vi "UHR-Fleezers Control (host) - Lorentz v4.vi"() -> ()   [LabVIEW 2014] (continued)
                n3907 = Array Subset(array=w6030, index=w5984, length="N pts to average") -> (w6046:dbl[])
                n3908 = Array Subset(array=w6025, index=w5983, length="N pts to average") -> (w6028:dbl[])
                n3909 = Array Subset(array=w6025, index=w5984, length="N pts to average") -> (w6027:dbl[])
                n3910 = Array Subset(array=w5986, index=w5983, length="N pts to average") -> (w5995:dbl[])
                n3911 = Array Subset(array=w5986, index=w5984, length="N pts to average") -> (w5994:dbl[])
                n3912 = Index Array(array=w6008, index=0) -> (element=w6006:waveform(dbl))
                n3913 = call-poly <vilib>:"Mean.vi"("X"=w6047) -> ("mean"=w6045:dbl)  [unwired: 1 out]
                n3914 = call-poly <vilib>:"Mean.vi"("X"=w6028) -> ("mean"=w6024:dbl)  [unwired: 1 out]
                n3915 = call-poly <vilib>:"Mean.vi"("X"=w6046) -> ("mean"=w6044:dbl)  [unwired: 1 out]
                n3916 = call-poly <vilib>:"Mean.vi"("X"=w6027) -> ("mean"=w6023:dbl)  [unwired: 1 out]
                n3917 = call-poly <vilib>:"Mean.vi"("X"=w5995) -> ("mean"=w5993:dbl)  [unwired: 1 out]
                n3918 = call-poly <vilib>:"Mean.vi"("X"=w5994) -> ("mean"=w5992:dbl)  [unwired: 1 out]
                n3919 = Unbundle By Name(w6006) -> ("Y"=w6004:dbl[])
                n3920 = Subtract(x=w6024, y=w6023) -> (x-y=w6015:dbl)
                "Delta Fl. 2" <- w6015
                n3921 = Subtract(x=w5993, y=w5992) -> (x-y=w5987:dbl)
                "Delta Fl. 3" <- w5987
                n3922 = Subtract(x=w6045, y=w6044) -> (x-y=w6042:dbl)
                "Delta Fl. 1" <- w6042
                n3923 = feedback #34(w6004) -> (w6003:dbl[])
                n3924 = Build Array (concatenate)(w6003, w6004) -> (w6005:dbl[])
                n3925 = Initialize Array(w6042, 1 ("dimension size")) -> (w6039:dbl[])
                n3926 = Initialize Array(w6015, 1 ("dimension size")) -> (w6020:dbl[])
                n3927 = Initialize Array(w5987, 1 ("dimension size")) -> (w5989:dbl[])
                n3928 = Select(t=w6004, s=w5975, f=w6005) -> (s? t:f=w6002:dbl[])
                "Saved trap pos" <- w6002
                n3929 = feedback-in #34(w6002) -> ()
                n3930 = feedback #35(w6039) -> (w6040:dbl[])
                n3931 = Build Array (concatenate)(w6040, w6039) -> (w6038:dbl[])
                n3932 = feedback #36(w6020) -> (w6021:dbl[])
                n3933 = feedback #37(w5989) -> (w5990:dbl[])
                n3934 = Build Array (concatenate)(w6021, w6020) -> (w6019:dbl[])
                n3935 = Build Array (concatenate)(w5990, w5989) -> (w5988:dbl[])
                n3936 = Select(t=w6039, s=w5975, f=w6038) -> (s? t:f=w6018:dbl[])
                n3937 = feedback-in #35(w6018) -> ()
                n3938 = Select(t=w6020, s=w5975, f=w6019) -> (s? t:f=w6017:dbl[])
                n3939 = feedback-in #36(w6017) -> ()
                n3940 = Select(t=w5989, s=w5975, f=w5988) -> (s? t:f=w5982:dbl[])
                n3941 = feedback-in #37(w5982) -> ()
                n3942 = Build Array(w6018, w6017, w5982) -> (→"Save APD Deriv":dbl[][])
                n3943 = Index Array(array=w5974, index=15) -> (element=w5980:waveform(dbl))
                n3944 = Unbundle By Name(w5980) -> ("Y"=w5978:dbl[])
                n3945 = feedback #38(w5978) -> (w5977:dbl[])
                n3946 = Build Array (concatenate)(w5977, w5978) -> (w5979:dbl[])
                n3947 = Select(t=w5978, s=w5975, f=w5979) -> (s? t:f=w5976:dbl[])
                "Amp current" <- w5976
                n3948 = feedback-in #38(w5976) -> ()
              }
            }
            "Progress" <- w5951
            "Progress 2" <- w5951
          }
        }
      }
    }
    n3949 = local read "wait to reset values"() -> (w4817:bool)
    n3950 = Not(x=w4815) -> (.not. x?=w4818:bool)
    n3951 = And(x=w4818, y=w4817) -> (x .and. y?=w4819:bool)
    n3952 = case "Part of MCL raster scanning: returns to initial positions after scan done" shown="True" w4819 {
      tunnel: w4565 -> [w5414 w5421]
      tunnel: [w5414 w5420] -> w4821
      tunnel: w4666 -> [w5413 w5419]
      tunnel: [w5413 w5418] -> w4816
      frame False {
      }
      frame True {
        w5429 = 10.0 ("y")
        w5428 = 32767.0 ("y")
        # "to return scan values\nafter a synchronous \nAOM scan"
        n3953 = local read "AO2"() -> (w5422:dbl)
        n3954 = local read "AO1"() -> (w5423:dbl)
        n3955 = local write "wait to reset values"(FALSE ("wait to reset values")) -> ()
        n3956 = Multiply(x=w5423, y=w5428) -> (x*y=w5425:dbl)
        n3957 = Multiply(x=w5422, y=w5428) -> (x*y=w5427:dbl)
        n3958 = Divide(x=w5425, y=w5429) -> (x/y=w5424:dbl)
        n3959 = Divide(x=w5427, y=w5429) -> (x/y=w5426:dbl)
        n3960 = To Word Integer(number=w5424) -> (16bit integer=w5430:i16)
        n3961 = To Word Integer(number=w5426) -> (16bit integer=w5431:i16)
        n3962 = local read "Total Counts (ticks)"() -> (w5415:u16)
        n3963 = local read "Scan Range (V)\n(of steps)"() -> (w5416:dbl)
        n3964 = xnode "Read/Write Control"("FPGA VI Reference In"=w5421, "error in"=w5419, "AO1"=w5430, "AO2"=w5431, "MCL count"=w5415) -> ("FPGA VI Reference Out"=w5420:T50, "error out"=w5418:errorcluster)
        n3965 = property on="Scan Range (V)\n(of steps)" class="DigNum (strict)"("Val(Sgnl)"=w5416) -> ()  [unwired: 2 in, 2 out]
      }
    }
    n3966 = case shown="True" "Sound ON" {
      tunnel: [w4934 w4979] -> w4618
      tunnel: w4617 -> [w4934 w4978]
      tunnel: w4615 -> [_ _]
      tunnel: w4594 -> [_ w4937]
      tunnel: w4614 -> [_ _]
      tunnel: w4613 -> [_ w4948]
      tunnel: w4612 -> [_ w4958]
      frame False {
      }
      frame True {
        n3967 = Index Array(array=w4937, index="Data channel to sound") -> (element=w4936:waveform(dbl))
        "Waveform Graph 2" <- w4936
        n3968 = Unbundle By Name(w4936) -> ("dt"=w4962:dbl, "Y"=w4960:dbl[])
        n3969 = Array Size(array=w4960) -> (size(s)=w4961:i32)
        "N data samples" <- w4961
        n3970 = for "Data time base" {
          N: w4961 -> [_]
          tunnel: [w4983] -> w4963 mode=indexing
          i -> [w4983]
        }
        n3971 = Multiply(x=w4962, y=w4963) -> (x*y=w4959:dbl[])
        n3972 = Compound Arithmetic op=MULTIPLY(6.283185307179586, "Carrier Frequency (Hz)", w4958) -> (w4975:dbl[])
        n3973 = call <vilib>:"Interpolate 1D.vi"("X is monotonic"=TRUE, "xi"=w4958, "X"=w4959, "Y"=w4960) -> ("yi"=w4956:dbl[])  [unwired: 5 in, 2 out]
        n3974 = Sine(x=w4975) -> (sin(x)=w4964:dbl[])
        n3975 = Add(x=w4956, y="Offset") -> (x+y=w4954:dbl[])
        n3976 = Multiply(x=w4954, y="mult x") -> (x*y=w4952:dbl[])
        n3977 = Add(x="Offset 2", y=w4952) -> (x+y=w4947:dbl[])
        n3978 = Compound Arithmetic op=MULTIPLY(6.283185307179586, "Carrier Frequency (Hz)", w4948, w4947) -> (w4939:dbl[])
        n3979 = for "Cumulative sum" {
          tunnel: [w4982] -> w4945 mode=indexing
          shift-right: [w4982] -> w4942
          shift-left: 0.0 -> [w4981]
          tunnel: w4939 -> [w4980] mode=indexing
          n3980 = Add(x=w4980, y=w4981) -> (x+y=w4982:dbl)
        }
        n3981 = feedback #39(0.0) -> (w4941:dbl)
        n3982 = Add(x=w4945, y=w4941) -> (x+y=w4944:dbl[])
        n3983 = Add(x=w4942, y=w4941) -> (x+y=w4940:dbl)
        n3984 = feedback-in #39(w4940) -> ()
        n3985 = Sine(x=w4944) -> (sin(x)=w4938:dbl[])
        n3986 = Select(t=w4964, s="tone or data", f=w4938) -> (s? t:f=w4970:dbl[])
        n3987 = Multiply(x=w4970, y="Volume") -> (x*y=w4968:dbl[])
        n3988 = Initialize Array(0.0 ("element"), "N initial buffer elements") -> (w4971:dbl[])
        n3989 = Multiply(x="N initial buffer elements", y=w4948) -> (x*y=→"Initial buffer time (s)":dbl)
        n3990 = Build Array (concatenate)(w4971, w4968) -> (w4973:dbl[])
        n3991 = First Call?() -> (First Call?: T/F=w4974:bool)
        n3992 = Select(t=w4973, s=w4974, f=w4968) -> (s? t:f=w4967:dbl[])
        n3993 = call-poly <vilib>:"Sound Output Write.vi"("data"=w4967, "task ID"=w4978) -> ("task ID out"=w4979:T60)  [unwired: 8 in, 1 out]
      }
    }
    n3994 = node-c288() -> ()  [unwired: 2 out]
  }
  n3995 = VISA Close(VISA resource name=w19) -> ()  [unwired: 1 in, 1 out]
  n3996 = disable-structure shown="Disabled" {
    disable-tunnel: w37 -> [w6119 _]
    frame Disabled {
      n3997 = call <vilib>:"Sound Output Clear.vi"("task ID"=w6119) -> ()  [unwired: 10 in, 1 out]
    }
    frame Enabled {
    }
  }
  n3998 = node-c288(w80) -> ()  [unwired: 1 out]
  n3999 = node-c288(w88) -> ()  [unwired: 1 out]
  n4000 = flat-sequence {
    tunnel: w95 -> [w6123]
    tunnel: w96 -> [w6124]
    tunnel: [w6122] -> w94
    tunnel: [w6121] -> w93
    tunnel: w92 -> [_]
    tunnel: w90 -> [_]
    tunnel: w86 -> [_]
    tunnel: w94 -> [w6125]
    tunnel: w93 -> [w6126]
    frame #0 {
      w6120 = FALSE ("AI to FIFO")
      n4001 = xnode "Read/Write Control"("FPGA VI Reference In"=w6124, "error in"=w6123, "AI to FIFO"=w6120, "APD to FIFO"=w6120) -> ("FPGA VI Reference Out"=w6122:T50, "error out"=w6121:errorcluster)
    }
    frame #1 {
      n4002 = xnode "Close FPGA VI Reference"("FPGA VI Reference In"=w6125, "error in"=w6126) -> ("error out"=→"error out":errorcluster)
    }
  }
